vi "Close Config File.vi"(8 "error in (no error)":errorcluster, 11 "file refnum":T1) -> (0 "error out":errorcluster, 3 "Path":path)   [LabVIEW 2019, in "TSC File IO.lvlib"]
doc: "This VI will close the configuration file.\n\nInputs:\n-file refnum [ref] - reference to the config file\n-error in\n\nOutputs:\n-Path [path] - a path to the file\n-error out\n\n<b>Code Developed By:</b>\nDaniel Coons\nTechnology Service Corporation\n1983 S Liberty Drive\nBloomington, IN 47403\nwww.tsc.com\\atcs"
uses:
  TSC File IO.lvlib
  <vilib>/Utility/config.llb/Config Data RefNum.ctl
  <vilib>/Utility/config.llb/NI_LVConfig.lvlib
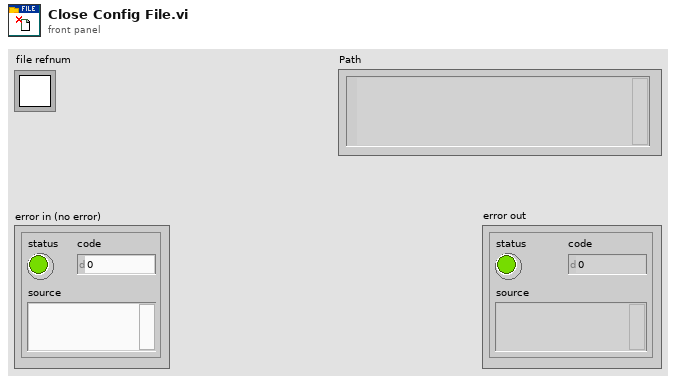
[diagram p1: front panel]
types:
  T1 = typedef "NI_LVConfig.lvlib/Config Data RefNum.ctl" = refnum<k1>
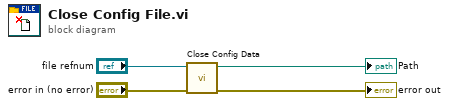
[diagram p0: block diagram]
diagram:
  n1 = call <vilib>:"Close Config Data.vi"("error in (no error)"="error in (no error)", "refnum"="file refnum") -> ("error out"=→"error out":errorcluster, "file path"=→"Path":path)  [unwired: 8 in]
